vi "Interpolation (SubVI).vi"(10 "Interpolation factor (n)":i32, 11 "Original Data (X,Y)":dbl[][](array[numeric])) -> (3 "Cluster":cluster{dbl[], dbl[]})   [LabVIEW 2017]
uses:
  <vilib>/Analysis/NI_AALPro.lvlib
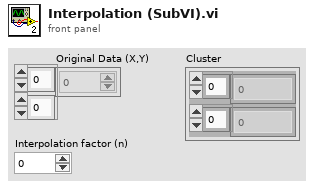
[diagram p1: front panel]
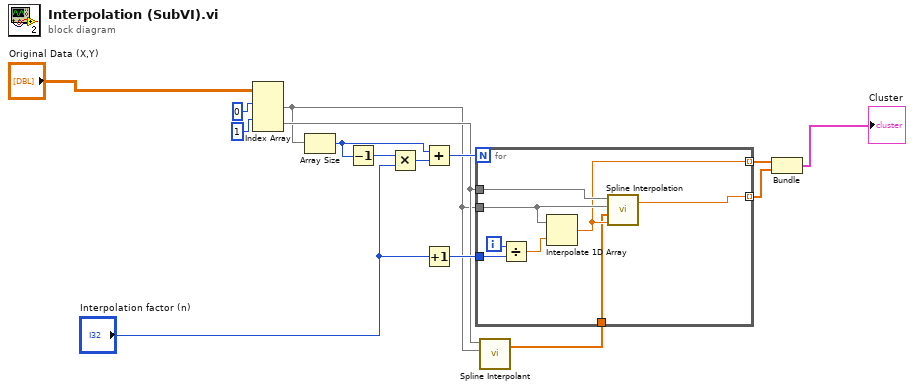
[diagram p0: block diagram]
diagram:
  n1 = Index Array(array="Original Data (X,Y)", index (row) #1=0, index (row) #2=1 ("index (col)")) -> (element #1=w2:dbl[], element #2=w3:dbl[])  [unwired: 2 in]
  n2 = Array Size(array=w2) -> (size(s)=w12:i32)
  n3 = Decrement(x=w12) -> (x-1=w9:i32)
  n4 = Multiply(x=w9, y="Interpolation factor (n)") -> (x*y=w11:i32)
  n5 = Add(x=w12, y=w11) -> (x+y=w13:i32)
  n6 = Increment(x="Interpolation factor (n)") -> (x+1=w10:i32)
  n7 = call <vilib>:"Spline Interpolant.vi"("X"=w2, "Y"=w3) -> ("Interpolant"=w1:dbl[])  [unwired: 2 in, 1 out]
  n8 = for {
    N: w13 -> [_]
    tunnel: w3 -> [w23]
    tunnel: w2 -> [w19]
    tunnel: w10 -> [w21]
    tunnel: [w20] -> w15 mode=indexing
    tunnel: [w18] -> w14 mode=indexing
    tunnel: w1 -> [w16]
    i -> [w22]
    n9 = Divide(x=w22, y=w21) -> (x/y=w17:dbl)
    n10 = Interpolate 1D Array(1:w17, 2:w19) -> (0:w18:dbl)
    n11 = call <vilib>:"Spline Interpolation.vi"("x value"=w18, "Interpolant"=w16, "X"=w19, "Y"=w23) -> ("interpolation value"=w20:dbl)  [unwired: 1 out]
  }
  n12 = Bundle(w14, w15) -> (→"Cluster":cluster{dbl[], dbl[]})  [unwired: 1 in]
